vi "Structured Light Code_fileversion.vi"() -> ()   [LabVIEW 2014]
panel:
  out "Input Image":T1(plugin-control)
  out "Final Output Image":T1(plugin-control)
  in  "stop":bool
  out "Running":bool
  in  "File Path":path
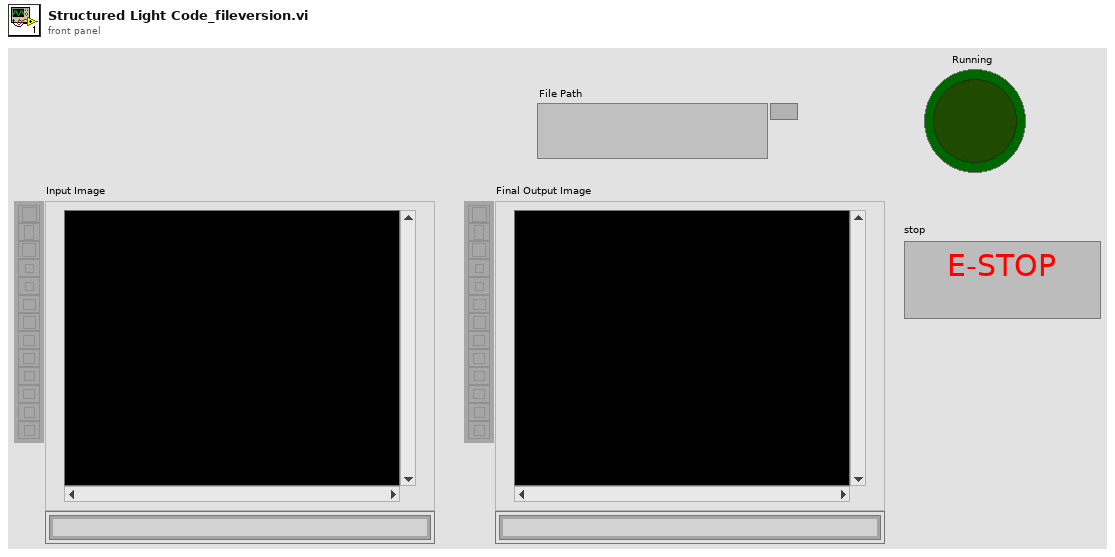
[diagram p1: front panel]
types:
  T1 = typedef "IMAQ Image.ctl" = refnum<image>
  T2 = typedef "Image Type" = u32
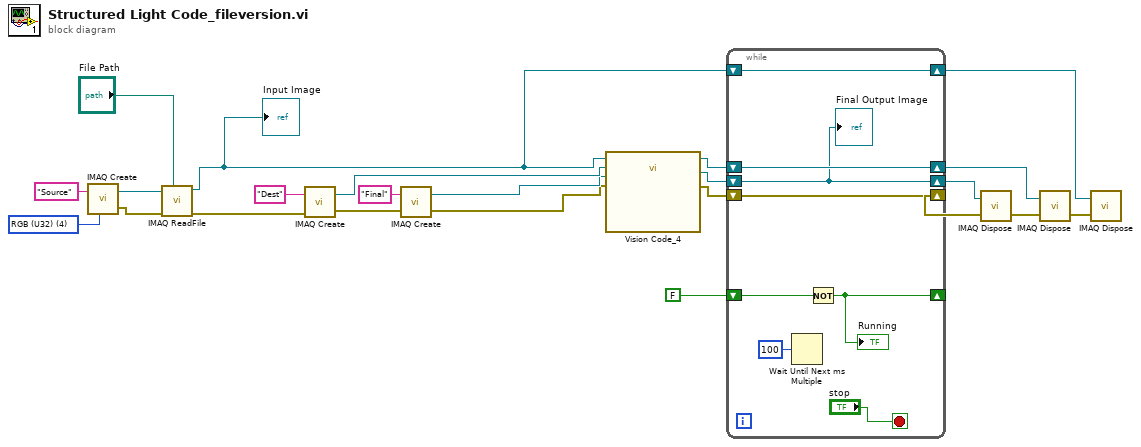
[diagram p0: block diagram]
diagram:
  w19 = T2 4 items=["Grayscale (U8)", "Grayscale (I16)", "Grayscale (SGL)", "Complex (CSG)", "RGB (U32)", "HSL (U32)", "RGB (U64)", "Grayscale (U16)"] ("Image Type")
  n1 = call "IMAQ Create"("Image Name"="Source", "Image Type"=w19) -> ("New Image"=w18:T1, "error out"=w17:errorcluster)  [unwired: 3 in]
  n2 = call "IMAQ ReadFile"("File Path"="File Path", "error in (no error)"=w17, "Image"=w18) -> ("error out"=w15:errorcluster, "Image Out"=w7:T1)  [unwired: 4 in, 3 out]
  "Input Image" <- w7
  n3 = call "IMAQ Create"("Image Name"="Dest", "error in (no error)"=w15) -> ("New Image"=w6:T1, "error out"=w22:errorcluster)  [unwired: 3 in]
  n4 = call "IMAQ Create"("Image Name"="Final", "error in (no error)"=w22) -> ("New Image"=w5:T1, "error out"=w4:errorcluster)  [unwired: 3 in]
  n5 = call "Vision Code_4.vi"("Image In"=w7, "Image Dst"=w6, "Final Image Output"=w5, "error in"=w4) -> ("Image Out"=w2:T1, "Output Image"=w1:T1, "error out"=w3:errorcluster)  [unwired: 21 in]
  n6 = while {
    shift-right: [w29] -> _
    shift-left: FALSE -> [w31]
    shift-right: [w25] -> w8
    shift-left: w7 -> [w25]
    shift-right: [w28] -> w9
    shift-left: w2 -> [w28]
    shift-right: [w26] -> w10
    shift-left: w1 -> [w26]
    shift-right: [w27] -> w11
    shift-left: w3 -> [w27]
    stop <- "stop" stop-if-true
    n7 = Wait Until Next ms Multiple(millisecond multiple=u32 100) -> ()  [unwired: 1 out]
    n8 = Not(x=w31) -> (.not. x?=w29:bool)
    "Running" <- w29
    "Final Output Image" <- w26
  }
  n9 = call "IMAQ Dispose"("Image"=w10, "error in (no error)"=w11) -> ("error out"=w14:errorcluster)  [unwired: 4 in]
  n10 = call "IMAQ Dispose"("Image"=w9, "error in (no error)"=w14) -> ("error out"=w13:errorcluster)  [unwired: 4 in]
  n11 = call "IMAQ Dispose"("Image"=w8, "error in (no error)"=w13) -> ()  [unwired: 4 in, 1 out]
